vi "incrementar_&checkfinal_traspaso.vi"(8 "error in (no error)":errorcluster, 10 "TRASPASO ASICS INPUT":T1={"COORD X ORIGEN"=0, "COORD  Y ORIGEN"=0, "NºASICS A MOVER"=1, "BANDEJA ORIGEN"=enum."BANDEJA ENTRADA", "BANDEJA DESTINO"=enum."BANDEJA ENTRADA", "COORD X DESTINO "=0, "COORD  Y DESTINO "=0, "CONTEO TRASLADOS"=0}) -> (0 "error out":errorcluster, 1 "FINAL ASICS??":bool, 2 "output cluster":T1={"COORD X ORIGEN"=0, "COORD  Y ORIGEN"=0, "NºASICS A MOVER"=1, "BANDEJA ORIGEN"=enum."BANDEJA ENTRADA", "BANDEJA DESTINO"=enum."BANDEJA ENTRADA", "COORD X DESTINO "=0, "COORD  Y DESTINO "=0, "CONTEO TRASLADOS"=0}, 3 "Asics pendientes":u32)   [LabVIEW 2019]
uses:
  TYPE'S DEF/INPUT_TRASPASO_ASICS.ctl
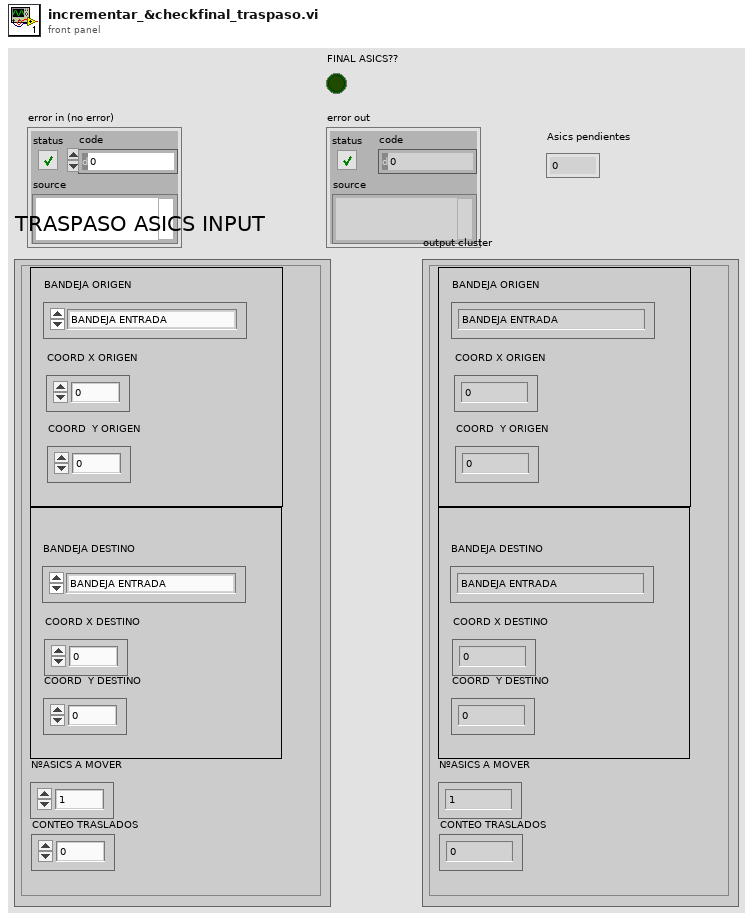
[diagram p1: front panel]
types:
  T1 = typedef "INPUT_TRASPASO_ASICS.ctl" = cluster{"COORD X ORIGEN":u32, "COORD  Y ORIGEN":u32, "NºASICS A MOVER":u32, "BANDEJA ORIGEN":enum16{"BANDEJA ENTRADA", "BANDEJA OK", "BANDEJA NOK"}, "BANDEJA DESTINO":enum16{"BANDEJA ENTRADA", "BANDEJA OK", "BANDEJA NOK"}, "COORD X DESTINO ":u32, "COORD  Y DESTINO ":u32, "CONTEO TRASLADOS":u32}
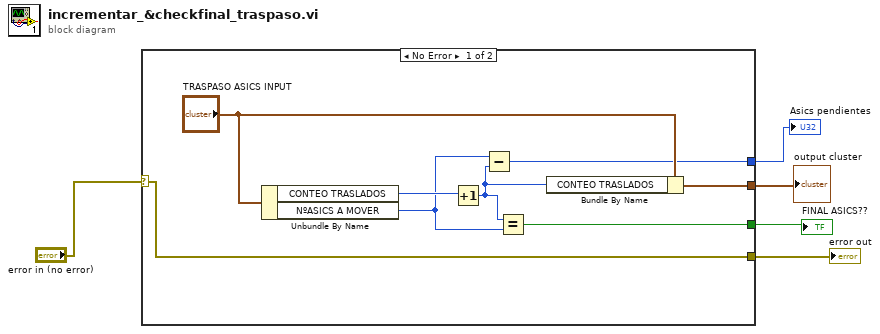
[diagram p0: block diagram]
diagram:
  n1 = case shown="No Error" "error in (no error)" {
    selector: "error in (no error)" -> [w8 w14]
    tunnel: [w9 _] -> w5
    tunnel: [w8 w14] -> w3
    tunnel: [w7 _] -> w2
    tunnel: [w6 _] -> w1
    frame No Error {
      n2 = Unbundle By Name("TRASPASO ASICS INPUT") -> ("CONTEO TRASLADOS"=w13:u32, "NºASICS A MOVER"=w11:u32)
      n3 = Increment(x=w13) -> (x+1=w12:u32)
      n4 = Subtract(x=w11, y=w12) -> (x-y=w6:u32)
      n5 = Equal?(x=w12, y=w11) -> (x = y?=w7:bool)
      n6 = Bundle By Name(cluster="TRASPASO ASICS INPUT", "CONTEO TRASLADOS"=w12) -> (w9:T1)
    }
    frame Error {
    }
  }
  "error out" <- w3
  "output cluster" <- w5
  "FINAL ASICS??" <- w2
  "Asics pendientes" <- w1
